vi "RDS Serial Config.vi"(8 "error in (no error)":errorcluster, 11 "RDS Serial Instrument Actor in":refnum<class "RDS Serial Instrument Actor.lvclass">) -> (0 "error out":errorcluster, 1 "baud rate (9600)":u32, 2 "VISA resource name":refnum<visa-resource-name>, 3 "RDS Serial Instrument Actor out":refnum<class "RDS Serial Instrument Actor.lvclass">, 5 "Termination Char(s)":string)   [LabVIEW 2015]
uses:
  RDS Serial Instrument Actor.lvclass
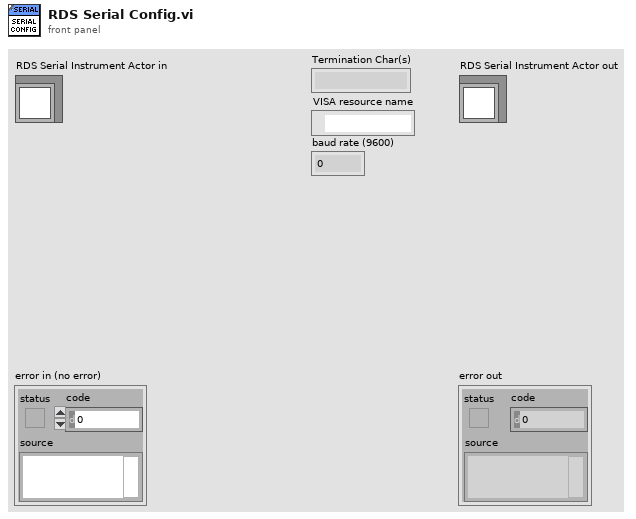
[diagram p1: front panel]
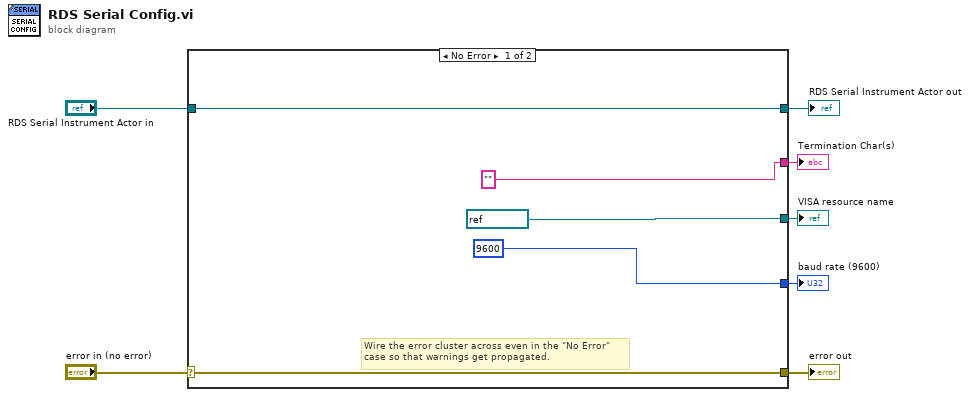
[diagram p0: block diagram]
diagram:
  n1 = case shown="No Error" "error in (no error)" {
    selector: "error in (no error)" -> [w11 w14]
    tunnel: [w11 w14] -> w6
    tunnel: [w12 w13] -> w4
    tunnel: "RDS Serial Instrument Actor in" -> [w12 w13]
    tunnel: ["" ("Termination Char(s)") _] -> w3
    tunnel: [refnum<visa-resource-name> "COM1" ("VISA resource name") _] -> w2
    tunnel: [u32 9600 ("baud rate (9600)") _] -> w1
    frame No Error {
      # "Wire the error cluster across even in the \"No Error\"\ncase so that warnings get propagated."
    }
    frame Error {
    }
  }
  "error out" <- w6
  "RDS Serial Instrument Actor out" <- w4
  "Termination Char(s)" <- w3
  "VISA resource name" <- w2
  "baud rate (9600)" <- w1
